vi "myRIO v1.0 AudioIn Block Read.vi"(6 "AudioIn FIFO Sample Rate":dbl=1000.0 min=1000.0 max=30000.0, 7 "Scale Constants Array":T1, 8 "error in (no error)":errorcluster, 9 "Number of Samples":u32=1000, 10 "AudioIn (N Samples) Channel List":T5, 11 "myRIO Ref In":T3) -> (0 "error out":errorcluster, 2 "dbl Scaled Value List":dbl[][](array[numeric]), 3 "myRIO Ref Out":T3)   [LabVIEW 2021]
uses:
  <vilib>/myRIO/Common/Instrument Driver Framework/myRIO v1.0/AudioIn Block/typedefs/AudioIn Block Channels List.ctl
  <vilib>/myRIO/Common/Instrument Driver Framework/myRIO v1.0/AudioIn Block/typedefs/AudioIn Block Channels Enum.ctl
  <vilib>/myRIO/Common/Instrument Driver Framework/Utilities/typedefs/myRIO v1.0 Reference.ctl
  <vilib>/myRIO/Common/Instrument Driver Framework/Utilities/typedefs/Generic FPGA Reference.ctl
  <vilib>/myRIO/Common/Instrument Driver Framework/Utilities/typedefs/Analog Scaling Constants List.ctl
  <vilib>/myRIO/Common/Instrument Driver Framework/Utilities/typedefs/Analog Scaling Constants.ctl
  <vilib>/myRIO/Common/Instrument Driver Framework/myRIO v1.0/AudioIn Block/typedefs/AudioIn Block Channels FPGA Reference.ctl
  <vilib>/myRIO/Common/Instrument Driver Framework/myRIO v1.0/Resource Manager/vis/myRIO v1.0 Block Write Configuration.vi
  <vilib>/rvi/errors/niLvFpgaAdjustHostInterfaceError.vi
  <vilib>/rvi/interface/nirviReadWriteControl/nirviReadWriteControl.xnode
  <vilib>/rvi/interface/nirviMethod/nirviMethod.xnode
  <vilib>/rvi/interface/Simulation/niFpgaSimulationCallBeginRW.vi
  <vilib>/rvi/errors/niLvFpgaMergeErrorWithErrorCode.vi
  NiFpgaLv.dll
  <vilib>/FPGAPlugInAG/Dynamic/niLvFpga_StartFifo_Dynamic.vi
  <vilib>/FPGAPlugInAG/Dynamic/niLvFpga_StopFifo_Dynamic.vi
  <vilib>/FPGAPlugInAG/Dynamic/niLvFpga_ReadFifo_Dynamic.vi
panel:
  # "This VI reads audio values from  user specified audio channels on\nthe myRIO v1.0 hardware. The values are read on the FPGA as u16 and \nscaled to dbl based on the specifications of the ADC. Please see Block Diagram for details."
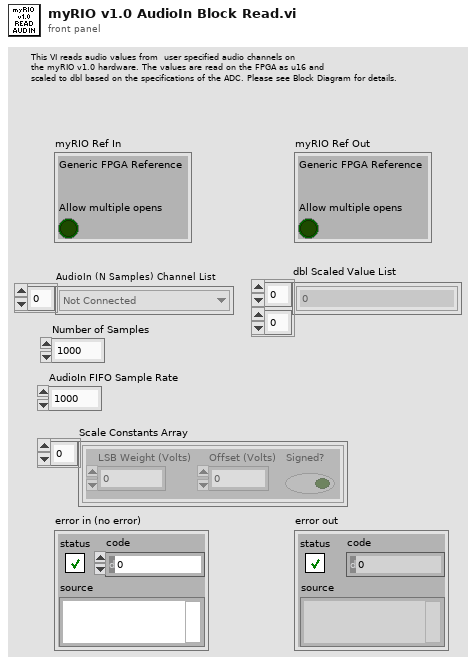
[diagram p1: front panel]
types:
  T1 = typedef "Analog Scaling Constants List.ctl" = T2[]
  T2 = typedef "Analog Scaling Constants.ctl" = cluster{"LSB Weight (Volts)":dbl, "Offset (Volts)":dbl, "Signed?":bool}
  T3 = typedef "myRIO v1.0 Reference.ctl" = cluster{"Generic FPGA Reference":T4, "Allow multiple opens":bool}
  T4 = typedef "Generic FPGA Reference.ctl" = refnum<k20>
  T5 = typedef "AudioIn Block Channels List.ctl" = T6[]
  T6 = typedef "AudioIn Block Channels Enum.ctl" = enum16{"Not Connected", "AudioIn/Left (N Samples)", "AudioIn/Right (N Samples)"}
  T7 = typedef "AudioIn Block Channels FPGA Reference.ctl" = refnum<k20>
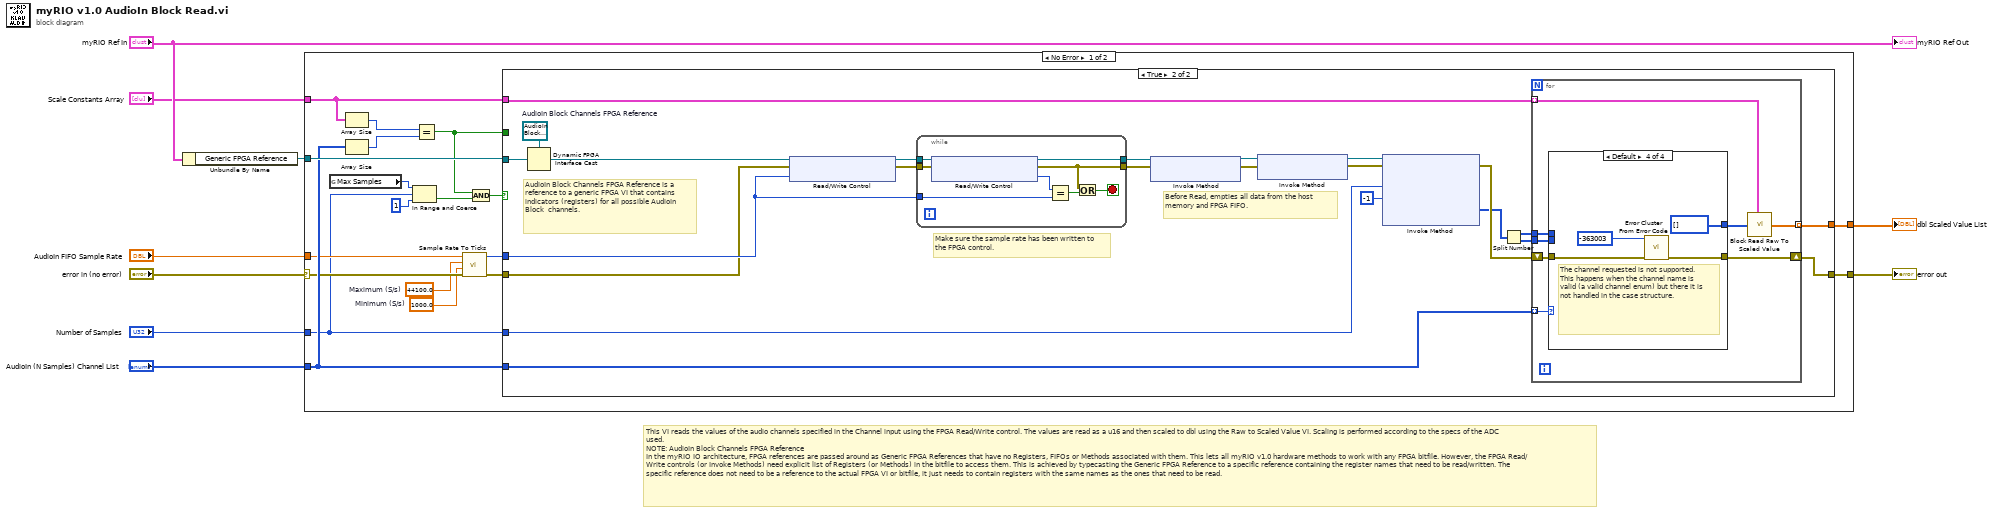
[diagram p0: block diagram]
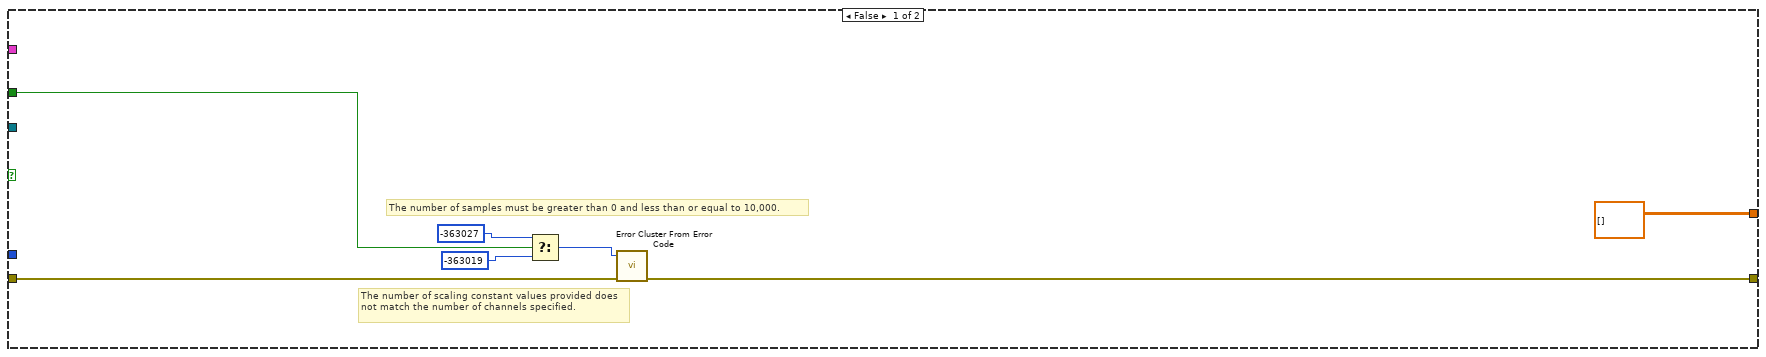
[diagram p2: hidden frame]
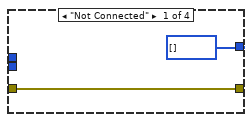
[diagram p3: hidden frame]
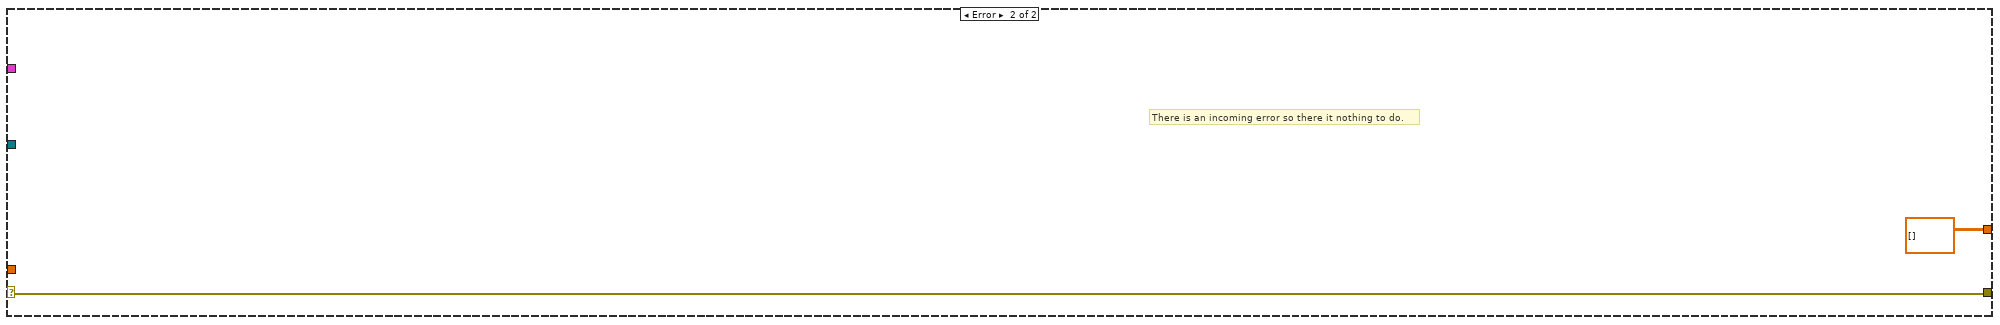
[diagram p6: hidden frame]
diagram:
  # "This VI reads the values of the audio channels specified in the Channel input using the FPGA Read/Write control. The values are read as a u16 and then scaled to dbl using the Raw to Scaled Value VI. Scaling is performed according to the specs of the ADC used.\nNOTE: AudioIn Block Channels FPGA Reference\nIn the myRIO IO architecture, FPGA references are passed around as Generic FPGA References that have no Registers, FIFOs or Methods associated with them. This lets all myRIO v1.0 hardware methods to work with any FPGA bitfile. However, the FPGA Read/Write controls (or Invoke Methods) need explicit list of Registers (or Methods) in the bitfile to access them. This is achieved by typecasting the Generic FPGA Reference to a specific reference containing the register names that need to be read/written. The specific reference does not need to be a reference to the actual FPGA VI or bitfile, it just needs to contain registers with the same names as the ones that need to be read."
  n1 = Unbundle By Name("myRIO Ref In") -> ("Generic FPGA Reference"=w5:T4)
  n2 = case shown="No Error" "error in (no error)" {
    selector: "error in (no error)" -> [w17 w86]
    tunnel: w5 -> [w28 _]
    tunnel: [w27 w86] -> w9
    tunnel: [w26 dbl[][] []] -> w8
    tunnel: "AudioIn (N Samples) Channel List" -> [w23 _]
    tunnel: "AudioIn FIFO Sample Rate" -> [w16 _]
    tunnel: "Number of Samples" -> [w13 _]
    tunnel: "Scale Constants Array" -> [w22 _]
    frame No Error {
      w14 = 1000.0  # Minimum (S/s)
      w15 = 44100.0  # Maximum (S/s)
      n3 = global read "myRIO v1.0 Block Write Configuration.vi" "Max Samples"() -> (w12:u32)
      n4 = Array Size(array=w22) -> (size(s)=w25:i32)
      n5 = Array Size(array=w23) -> (size(s)=w24:i32)
      n6 = In Range and Coerce(upper limit=w12, x=w13, lower limit=u32 1) -> (In Range?=w10:bool)  [unwired: 1 out]
      n7 = Equal?(x=w25, y=w24) -> (x = y?=w20:bool)
      n8 = call <vilib>:"Sample Rate To Ticks.vi"("error in (no error)"=w17, "Minimum (S/s)"=w14, "Maximum (S/s)"=w15, "Sample Rate (S/s)"=w16) -> ("error out"=w18:errorcluster, "Count (tick/s)"=w19:u32)  [unwired: 5 in, 1 out]
      n9 = And(x=w20, y=w10) -> (x .and. y?=w21:bool)
      n10 = case shown="True" w21 {
        tunnel: w28 -> [_ w58]
        tunnel: [w34 w57] -> w27
        tunnel: [dbl[][] [] ("dbl Scaled Value") w56] -> w26
        tunnel: w19 -> [_ w49]
        tunnel: w13 -> [_ w39]
        tunnel: w18 -> [w35 w48]
        tunnel: w23 -> [_ w54]
        tunnel: w22 -> [_ w53]
        tunnel: w20 -> [w32 _]
        frame False {
          # "The number of samples must be greater than 0 and less than or equal to 10,000."
          # "The number of scaling constant values provided does not match the number of channels specified."
          n11 = Select(t=-363027 ("error code (0)"), s=w32, f=-363019 ("error code (0)")) -> (s? t:f=w29:i32)
          n12 = call <vilib>:"Error Cluster From Error Code.vi"("error in (no error)"=w35, "error code (0)"=w29) -> ("error out"=w34:errorcluster)  [unwired: 7 in]
        }
        frame True {
          w55 = T7 refnum  # AudioIn Block Channels FPGA Reference
          # "Make sure the sample rate has been written to the FPGA control."
          # "Before Read, empties all data from the host memory and FPGA FIFO."
          # "AudioIn Block Channels FPGA Reference is a reference to a generic FPGA VI that contains indicators (registers) for all possible AudioIn Block  channels."
          n13 = Dynamic FPGA Interface Cast(Session In=w55, Type=w58) -> (Session Out=w50:T7)
          n14 = xnode "Read/Write Control"("FPGA VI Reference In"=w50, "error in"=w48, "AI.AudioIn.SampleRate"=w49) -> ("FPGA VI Reference Out"=w46:T7, "error out"=w47:errorcluster)
          n15 = while {
            tunnel: w46 -> [w63]
            tunnel: w47 -> [w62]
            tunnel: [w59] -> w45
            tunnel: [w60] -> w37
            tunnel: w49 -> [w66]
            stop <- w64 stop-if-true
            n16 = xnode "Read/Write Control"("FPGA VI Reference In"=w63, "error in"=w62) -> ("FPGA VI Reference Out"=w59:T7, "error out"=w60:errorcluster, "AI.AudioIn.SampleRate"=w61:u32)
            n17 = Equal?(x=w61, y=w66) -> (x = y?=w65:bool)
            n18 = Or(x=w60, y=w65) -> (x .or. y?=w64:bool)
          }
          n19 = xnode "Invoke Method"("FPGA VI Reference In"=w45, "error in"=w37) -> ("FPGA VI Reference Out"=w43:T7, "error out"=w42:errorcluster)
          n20 = xnode "Invoke Method"("FPGA VI Reference In"=w43, "error in"=w42) -> ("FPGA VI Reference Out"=w44:T7, "error out"=w41:errorcluster)
          n21 = xnode "Invoke Method"("FPGA VI Reference In"=w44, "error in"=w41, "Number of Elements"=w39, "Timeout (ms)"=-1) -> ("error out"=w38:errorcluster, "Data"=w36:u32[])  [unwired: 2 out]
          n22 = Split Number(x=w36) -> (hi(x)=w52:u16[], lo(x)=w51:u16[])
          n23 = for {
            shift-right: [w73] -> w57
            shift-left: w38 -> [w74]
            tunnel: w54 -> [w72] mode=indexing
            tunnel: [w71] -> w56 mode=indexing
            tunnel: w52 -> [w70]
            tunnel: w53 -> [w68] mode=indexing
            tunnel: w51 -> [w67]
            n24 = case shown="Default" w72 {
              tunnel: w74 -> [w76 w78 w80 w82]
              tunnel: [w76 w78 w80 w83] -> w73
              tunnel: [u16[] [] w77 w79 u16[] []] -> w69
              tunnel: w70 -> [_ w77 _ _]
              tunnel: w67 -> [_ _ w79 _]
              frame "Not Connected" {
              }
              frame "AudioIn/Left (N Samples)" {
              }
              frame "AudioIn/Right (N Samples)" {
              }
              frame Default {
                # "The channel requested is not supported. This happens when the channel name is valid (a valid channel enum) but there it is not handled in the case structure."
                n25 = call <vilib>:"Error Cluster From Error Code.vi"("error in (no error)"=w82, "error code (0)"=-363003) -> ("error out"=w83:errorcluster)  [unwired: 7 in]
              }
            }
            n26 = call <vilib>:"Block Read Raw To Scaled Value.vi"("Scaling Constants"=w68, "u16 Raw Value"=w69) -> ("dbl Scaled Value"=w71:dbl[])  [unwired: 7 in]
          }
        }
      }
    }
    frame Error {
      # "There is an incoming error so there it nothing to do."
    }
  }
  "error out" <- w9
  "dbl Scaled Value List" <- w8
  "myRIO Ref Out" <- "myRIO Ref In"
